vi "Get Random Word.vi"() -> (3 "element":string)   [LabVIEW 2015]
uses:
  <vilib>/Utility/file.llb/Read Delimited Spreadsheet (string).vi
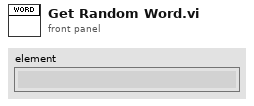
[diagram p1: front panel]
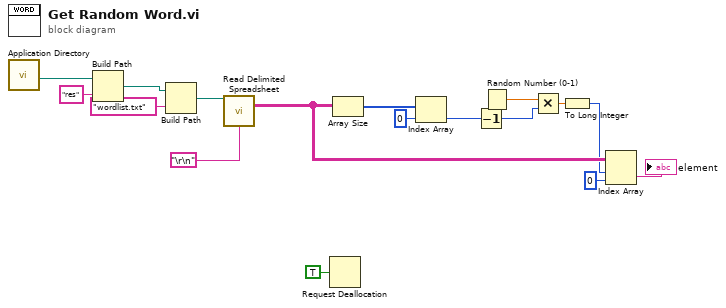
[diagram p0: block diagram]
diagram:
  n1 = call <vilib>:"Application Directory.vi"() -> ("Application Directory"=w17:path)
  n2 = Build Path(base path=w17, name or relative path="res") -> (appended path=w15:path)
  n3 = Build Path(base path=w15, name or relative path="wordlist.txt") -> (appended path=w13:path)
  n4 = call-poly <vilib>:"Read Delimited Spreadsheet.vi"("file path (dialog if empty)"=w13, "delimiter (\\t)"="\r\n") -> ("all rows"=w6:string[][])  [unwired: 8 in, 5 out]
  n5 = Request Deallocation(TRUE ("flag")) -> ()
  n6 = Array Size(array=w6) -> (size(s)=w11:i32[])
  n7 = Index Array(array=w11, index=0) -> (element=w8:i32)
  n8 = Decrement(x=w8) -> (x-1=w7:i32)
  n9 = Random Number (0-1)() -> (number: 0 to 1=w9:dbl)
  n10 = Multiply(x=w9, y=w7) -> (x*y=w4:dbl)
  n11 = To Long Integer(number=w4) -> (32bit integer=w3:i32)
  n12 = Index Array(array=w6, index (row)=w3, index (col)=0 ("disabled index (col)")) -> (element=→"element":string)
